vi "parse hex string.vi"(1 "hex string":string) -> (0 "data":u8[](array[numeric]))   [LabVIEW 2019, in "WebSocket Server Toolkit.lvlib"]
uses:
  WebSocket Server Toolkit.lvlib
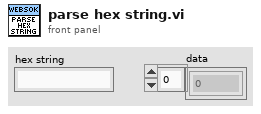
[diagram p1: front panel]
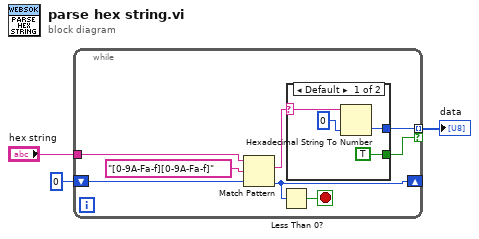
[diagram p0: block diagram]
diagram:
  n1 = while {
    tunnel: "hex string" -> [w11]
    shift-right: [w7] -> _
    shift-left: 0 ("offset (0)") -> [w9]
    tunnel: [w5] -> w3 mode=indexing if=w4
    stop <- w6 stop-if-true
    n2 = Match Pattern(string=w11, regular expression="[0-9A-Fa-f][0-9A-Fa-f]", offset (0)=w9) -> (match substring=w8:string, offset past match=w7:i32)  [unwired: 2 out]
    n3 = Less Than 0?(x=w7) -> (x < 0?=w6:bool)
    n4 = case shown="Default" w8 {
      selector: w8 -> [w15 _]
      tunnel: [w13 _] -> w5
      tunnel: [TRUE _] -> w4
      frame Default {
        n5 = Hexadecimal String To Number(string=w15, default (0uL)=u8 0 ("default (0 U32)")) -> (number=w13:u8)  [unwired: 1 in, 1 out]
      }
      frame "" {
      }
    }
  }
  "data" <- w3
